vi "Get Max Angle.vi"() -> ()   [LabVIEW 2014]
uses:
  Begin/Global RefNums.vi
  _Dependencies/NavX/navX-MXP IMU.lvlib
panel:
  out "Min Pitch":dbl
  out "Min Roll":dbl
  out "Max Roll":dbl
  out "Max Pitch":dbl
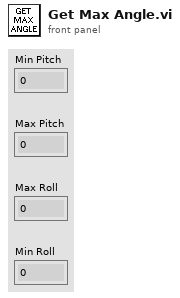
[diagram p1: front panel]
types:
  T1 = typedef "navX-MXP IMU.lvlib/navX Device TypeDef.ctl" = cluster{"navX Interface Protocol":T2, "navX Interface Protocol TypeDefs":cluster{"SPIDevRef":T3, "I2CDevRef":T6}, "navX System Information":cluster{"Board Information":T8, "Status":T9, "Offsets":T13}, "navX Common Information":cluster{"Update Rate (4Hz-60Hz)":T14, "refnum name":string, "error":errorcluster}}
  T2 = typedef "navX-MXP IMU.lvlib/navX Interface Protocol.ctl" = enum16{"SPI", "I2C"}
  T3 = typedef "WPI_SPIDevRef.ctl" = cluster{"DevStatus":errorcluster, "Handle":i32, "Controller":T4, "SPI Bus":T5}
  T4 = typedef "FPGA_TypedefDigitalModule.ctl" = enum16{"Controller 1"}
  T5 = typedef "spi_bus.ctl" = enum16{"SPI On-Board, CS0", "SPI On-Board, CS1", "SPI On-Board, CS2", "SPI On-Board, CS3", "SPI MXP", "Invalid"}
  T6 = typedef "WPI_I2CDevRef.ctl" = cluster{"DevStatus":errorcluster, "Controller":T4, "Device Address":u8, "Handle":i32, "I2C Bus":T7}
  T7 = typedef "i2c_bus.ctl" = enum16{"I2C On-Board", "I2C MXP", "Invalid"}
  T8 = typedef "navX-MXP IMU.lvlib/navX Board Information.ctl" = cluster{"WhoAmI (50 | 0x32)":u8, "Board Revision":u8, "Firmware Major Version":u8, "Firmware Minor Version":u8}
  T9 = typedef "navX-MXP IMU.lvlib/navX Status Data.ctl" = cluster{"Update Rate Hz":u8, "Accelerometer Full-Scale Range":u8, "Gyro Full-Scale Range":u16, "NAVX_OP_STATUS":T10, "NAVX_CAL_STATUS":T11, "NAVX_SELFTEST_STATUS":u8, "NAVX_SENSOR_STATUS":T12}
  T10 = typedef "navX-MXP IMU.lvlib/navX NAVX_OP_STATUS.ctl" = u8
  T11 = typedef "navX-MXP IMU.lvlib/navX NAVX_CAL_STATUS.ctl" = u8
  T12 = typedef "navX-MXP IMU.lvlib/navX NAVX_SENSOR_STATUS.ctl" = cluster{"MOVING":bool, "YAW_STABLE":bool, "MAG_DISTURBANCE":bool, "ALTITUDE_VALID":bool, "SEALEVEL_PRESS_SET":bool, "FUSED_HEADING_VALID":bool}
  T13 = typedef "navX-MXP IMU.lvlib/navX Offsets Data.ctl" = cluster{"Yaw":dbl, "Quat W":dbl, "Quat X":dbl, "Quat Y":dbl, "Quat Z":dbl}
  T14 = typedef "navX-MXP IMU.lvlib/navX Update Rate.ctl" = u8
  T15 = typedef "navX-MXP IMU.lvlib/navX YPRH Data.ctl" = cluster{"Yaw":dbl, "Pitch":dbl, "Roll":dbl, "Heading":dbl}
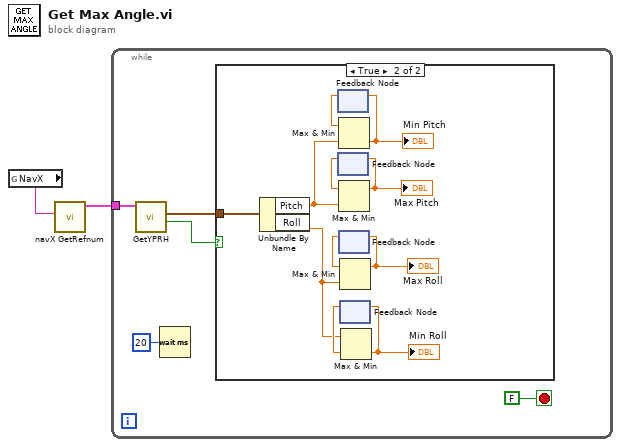
[diagram p0: block diagram]
diagram:
  n1 = global read "Global RefNums.vi" "NavX"() -> (w2:string)
  n2 = call "navX GetRefnum.vi"("refnum name"=w2) -> ("navX Device TypeDef"=w1:T1)  [unwired: 9 in, 1 out]
  n3 = while {
    tunnel: w1 -> [w5]
    stop <- FALSE stop-if-true
    n4 = call "GetYPRH.vi"("navX Device TypeDef"=w5) -> ("Valid?"=w3:bool, "YPRH"=w4:T15)  [unwired: 8 in, 1 out]
    n5 = Wait (ms)(milliseconds to wait=u32 20) -> ()  [unwired: 1 out]
    n6 = case shown="True" w3 {
      tunnel: w4 -> [_ w10]
      frame False {
      }
      frame True {
        n7 = Unbundle By Name(w10) -> ("Pitch"=w9:dbl, "Roll"=w8:dbl)
        n8 = feedback #1() -> (w12:dbl)  [unwired: 1 in]
        n9 = feedback #2() -> (w17:dbl)  [unwired: 1 in]
        n10 = Max & Min(x=w12, y=w9) -> (min(x,y)=w11:dbl)  [unwired: 1 out]
        "Min Pitch" <- w11
        n11 = feedback-in #1(w11) -> ()
        n12 = Max & Min(x=w17, y=w9) -> (max(x,y)=w18:dbl)  [unwired: 1 out]
        "Max Pitch" <- w18
        n13 = feedback-in #2(w18) -> ()
        n14 = feedback #3() -> (w16:dbl)  [unwired: 1 in]
        n15 = Max & Min(x=w16, y=w8) -> (max(x,y)=w15:dbl)  [unwired: 1 out]
        "Max Roll" <- w15
        n16 = feedback-in #3(w15) -> ()
        n17 = feedback #4() -> (w14:dbl)  [unwired: 1 in]
        n18 = Max & Min(x=w8, y=w14) -> (min(x,y)=w13:dbl)  [unwired: 1 out]
        "Min Roll" <- w13
        n19 = feedback-in #4(w13) -> ()
      }
    }
  }
